vi "_Database Driver Catalog.vi"   [LabVIEW 2014, in "hse-db.lvlib" / "ADO-DB-Driver.lvlib"]
uses:
  ADO-DB-Driver.lvlib
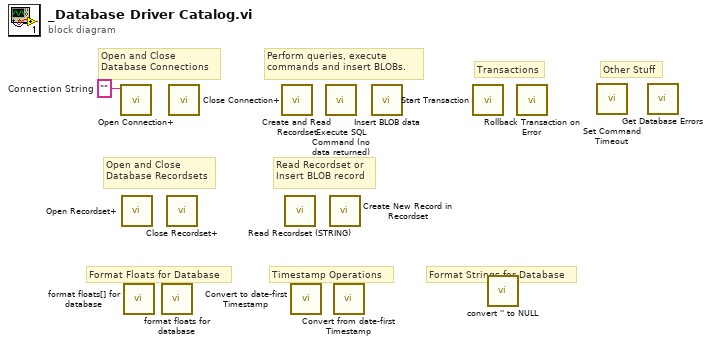
[diagram p0: block diagram]
diagram:
  w1 = ""  # Connection String
  # "Format Strings for Database"
  # "Timestamp Operations"
  # "Format Floats for Database"
  # "Read Recordset or\nInsert BLOB record"
  # "Open and Close\nDatabase Recordsets"
  # "Other Stuff"
  # "Transactions"
  # "Perform queries, execute\ncommands and insert BLOBs."
  # "Open and Close\nDatabase Connections"
  n1 = call "Open Connection+.vi"("Connection String"=w1) -> ()  [unwired: 8 in, 3 out]
  n2 = call "Open Recordset+.vi"() -> ()  [unwired: 10 in, 2 out]
  n3 = call "format floats[] for database.vi"() -> ()  [unwired: 5 in, 1 out]
  n4 = call "format floats for database.vi"() -> ()  [unwired: 5 in, 1 out]
  n5 = call "Close Recordset+.vi"() -> ()  [unwired: 11 in, 1 out]
  n6 = call "Close Connection+.vi"() -> ()  [unwired: 7 in, 1 out]
  n7 = call "Create and Read Recordset.vi"() -> ()  [unwired: 7 in, 5 out]
  n8 = call "Read Recordset (STRING).vi"() -> ()  [unwired: 7 in, 5 out]
  n9 = call "Convert to date-first Timestamp.vi"() -> ()  [unwired: 5 in, 1 out]
  n10 = call "Execute SQL Command (no data returned).vi"() -> ()  [unwired: 5 in, 3 out]
  n11 = call "Create New Record in Recordset.vi"() -> ()  [unwired: 8 in, 2 out]
  n12 = call "Convert from date-first Timestamp.vi"() -> ()  [unwired: 5 in, 1 out]
  n13 = call "Insert BLOB data.vi"() -> ()  [unwired: 8 in, 2 out]
  n14 = call "Start Transaction.vi"() -> ()  [unwired: 6 in, 2 out]
  n15 = call "convert '' to NULL.vi"() -> ()  [unwired: 5 in, 1 out]
  n16 = call "Rollback Transaction on Error.vi"() -> ()  [unwired: 9 in, 2 out]
  n17 = call "Set Command Timeout.vi"() -> ()  [unwired: 6 in, 2 out]
  n18 = call "Get Database Errors.vi"() -> ()  [unwired: 8 in, 2 out]
